vi "Test Code.vi"   [LabVIEW 2023]
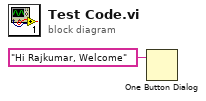
[diagram p0: block diagram]
diagram:
  n1 = One Button Dialog(message="Hi Rajkumar, Welcome") -> ()  [unwired: 1 in, 1 out]
